vi "Get_Frame_No.vi"(11 "Image In":T1) -> (3 "Frame Number":u32)   [LabVIEW 2015]
doc: "Use this template to build a VI to use as a subVI."
uses:
  <vilib>/vision/Image Controls.llb/IMAQ Image.ctl
  <vilib>/vision/NI_Vision_Development_Module.lvlib
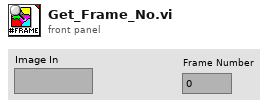
[diagram p1: front panel]
types:
  T1 = typedef "IMAQ Image.ctl" = refnum<image>
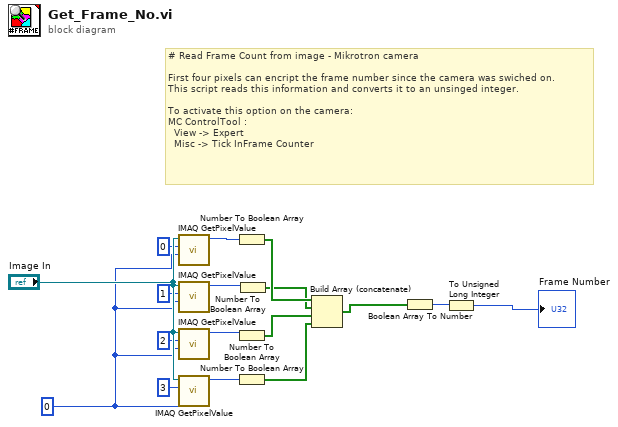
[diagram p0: block diagram]
diagram:
  w12 = 0 ("Y Coordinate")
  # "# Read Frame Count from image - Mikrotron camera\n\nFirst four pixels can encript the frame number since the camera was swiched on. \nThis script reads this information and converts it to an unsinged integer.\n\nTo activate this option on the camera:\nMC ControlTool :\n  View -> Expert\n  Misc -> Tick InFrame Counter"
  n1 = call "IMAQ GetPixelValue"("Image"="Image In", "X Coordinate"=0, "Y Coordinate"=w12) -> ("Pixel Value (U8)"=w11:u8)  [unwired: 3 in, 4 out]
  n2 = call "IMAQ GetPixelValue"("Image"="Image In", "X Coordinate"=1, "Y Coordinate"=w12) -> ("Pixel Value (U8)"=w7:u8)  [unwired: 3 in, 4 out]
  n3 = call "IMAQ GetPixelValue"("Image"="Image In", "X Coordinate"=2, "Y Coordinate"=w12) -> ("Pixel Value (U8)"=w8:u8)  [unwired: 3 in, 4 out]
  n4 = call "IMAQ GetPixelValue"("Image"="Image In", "X Coordinate"=3, "Y Coordinate"=w12) -> ("Pixel Value (U8)"=w9:u8)  [unwired: 3 in, 4 out]
  n5 = Number To Boolean Array(number=w11) -> (Boolean array=w6:bool[])
  n6 = Number To Boolean Array(number=w8) -> (Boolean array=w4:bool[])
  n7 = Number To Boolean Array(number=w9) -> (Boolean array=w3:bool[])
  n8 = Number To Boolean Array(number=w7) -> (Boolean array=w5:bool[])
  n9 = Build Array (concatenate)(w6, w5, w4, w3) -> (w2:bool[])
  n10 = Boolean Array To Number(Boolean array=w2) -> (number=w10:u32)
  n11 = To Unsigned Long Integer(number=w10) -> (unsigned 32bit integer=→"Frame Number":u32)
